vi "PH_PILS.set PPPA.vi"(0 "i ref in":refnum<vi>, 2 "Tagname":string="N/A", 5 "error in":errorcluster) -> (14 "i ref out":refnum<vi>, 19 "error out":errorcluster)   [LabVIEW 2014, in "PH_PILS.lvlib"]
uses:
  PH_PILS.lvlib
  PH_Basics/PH_PP_Common/PH_PP_Common.PUs.ctl
  PH_Basics/PH_PP_Common/PH_PP_Common.PSU Tags.ctl
  PH_Devices/PH_Beckhoff_PP_PU/PH_Beckhoff_PP_PU.RR Tags.ctl
  PH_Basics/PH_Common/PH_Common.lvlib
  PH_Basics/PH_PP_Common/PH_PP_Common.lvlib
  PH_Devices/PH_Beckhoff_PP_PU/PH_Beckhoff_PP_PU.lvlib
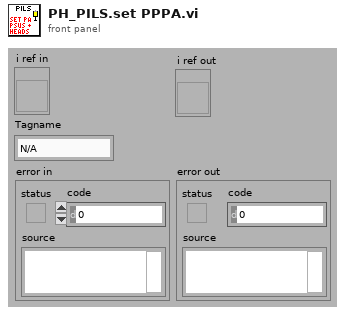
[diagram p1: front panel]
types:
  T1 = typedef "PH_PP_Common.lvlib/PH_PP_Common.PUs.ctl" = enum16{"no Info", "PA-19mm-1", "PA-19mm-2", "PA-45mm-PILC", "PA-45mm-MAIN", "MA-PU-1", "MA-PU-2", "MA-PU-3", "MA-PU-4", "MA-PU-5", "MA-PU-6", "MA-FR", "MA-PILC", "PA-45mm-DP"}
  T2 = typedef "PH_Beckhoff_PP_PU.lvlib/PH_Beckhoff_PP_PU.RR Tags.ctl" = enum16{"open", "closed", "close", "Status"}
  T3 = typedef "PH_PP_Common.lvlib/PH_PP_Common.PSU Tags.ctl" = enum16{"voltage-indicator", "peak-detect", "current", "voltage", "inihibit-indicator", "end-of-charge", "HV-on-indicator", "overtemperature", "interlock-indicator", "load-fault", "sum-fault", "HV-off-indicator", "DC-ok", "inhibit", "HV-on", "interlock", "reset", "Status", "Limits"}
  T4 = typedef "PH_PILS.lvlib/PH_PILS.i attribute.ctl" = cluster{"Boolean":cluster{"GUI Ref":refnum<vi>, "Status":i32}[], "GUI Refs Exp. Shutters":cluster{"1":refnum<vi>, "2":refnum<vi>, "3":refnum<vi>, "4":refnum<vi>}, "Tristate2Run GUI Refs":refnum<vi>[], "EO-Likes":cluster{"GUI Ref":refnum<vi>, "Status":i32}[], "Operation Mode":cluster{"Operation Mode":T5, "GUI":cluster{"Ref State":refnum<vi>, "Ref":refnum<vi>}, "Servicemode":cluster{"Tagname":string, "Status":i32}, "Labormode":cluster{"Tagname":string, "Status":i32}, "Searchmode":cluster{"Tagname":string, "Status":i32}, "Shotmode":cluster{"Tagname":string, "Status":i32}}, "Submode":cluster{"Submode":T6, "GUI":cluster{"Ref State":refnum<vi>, "Ref":refnum<vi>}, "Submode":cluster{"Tagname":string, "Status":i32}}, "Experiment":cluster{"Experiment":enum16{"unknown", "intern", "4 (Z6)", "3", "2", "1"}, "GUI":cluster{"Ref State":refnum<vi>, "Ref":refnum<vi>}, "intern":cluster{"Tagname":string, "Status":i32}, "Exp 4":cluster{"Tagname":string, "Status":i32}, "Exp 3":cluster{"Tagname":string, "Status":i32}, "Exp 2":cluster{"Tagname":string, "Status":i32}, "Exp 1":cluster{"Tagname":string, "Status":i32}}, "TristateNormal":cluster{"GUI Ref":refnum<vi>, "Status":i32}[], "Door Tags":cluster{"GUI Ref":refnum<vi>, "Status":i32}[], "GUIlessTags":cluster{"Name":string, "Status":i32}[], "Beamline GUI Refs":refnum<vi>[], "Special Boolean":cluster{"GUI Ref":refnum<vi>, "Status":i32}[], "Laserpower":cluster{"GUI Ref":refnum<vi>, "Status":i32}[], "Shutter":cluster{"GUI Ref":refnum<vi>, "Status":i32}[], "Tristate EO Like":cluster{"GUI Ref":refnum<vi>, "Status":i32}[], "PP":cluster{"GUI Ref":refnum<vi>, "Status":i32, "Head Ref":refnum<vi>, "Slider Ref":refnum<vi>}[], "Switch Knobs":cluster{"GUI Ref":refnum<vi>, "Status":i32}[], "Latch Knob GUI Refs":refnum<vi>[], "FailureCounter":i32, "Enabled Status":cluster{"Laser":i32, "PreAmp":i32, "MainAmp":i32}, "Mercury":refnum<vi>, "Instance Rods":string, "Logfile":path, "Beckhoff-Instance Internal":string, "Beckhoff-Instance External":string, "Enabling Rights":cluster{"Name":string, "Password":string, "PA?":bool, "MA?":bool, "Exp?":bool}[]}
  T5 = typedef "PH_PILS.lvlib/PH_PILS.Operation Mode.ctl" = enum16{"unknown", "Service", "Labor", "Search", "Shot"}
  T6 = typedef "PH_PILS.lvlib/PH_PILS.Submode.ctl" = enum16{"unknown", "HV-Normal", "HV-Test"}
  T7 = cluster{"GUI Ref":refnum<vi>, "Status":i32, "Head Ref":refnum<vi>, "Slider Ref":refnum<vi>}[]
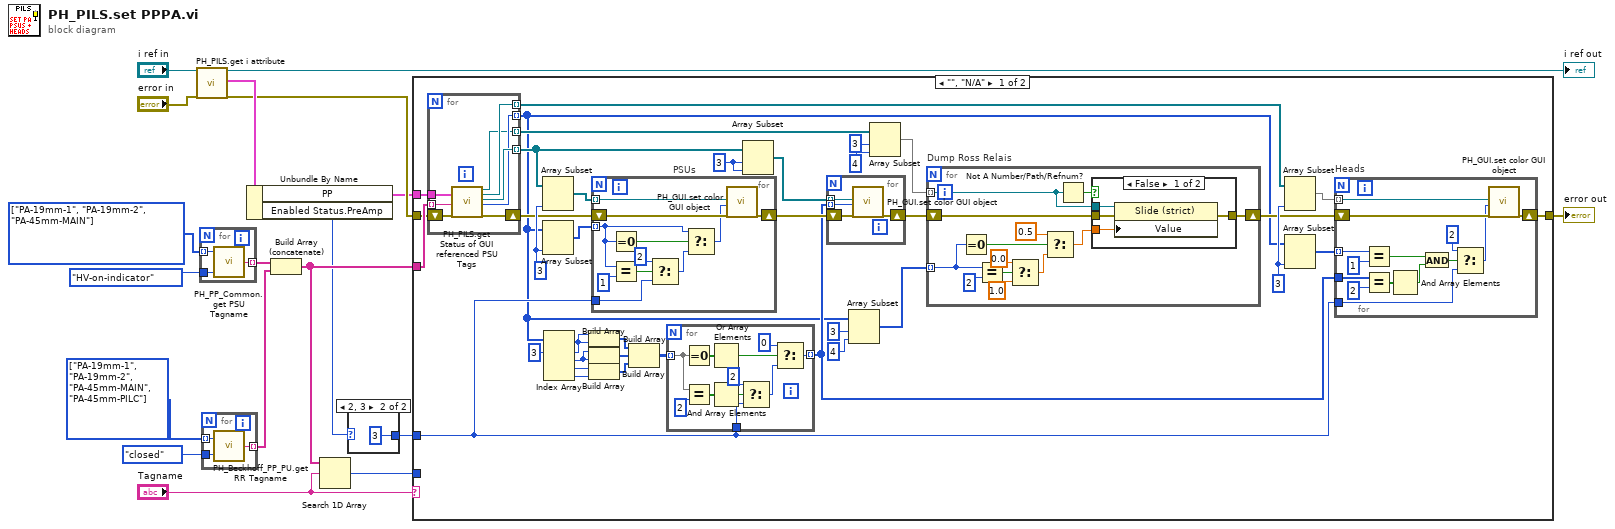
[diagram p0: block diagram]
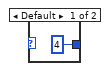
[diagram p2: hidden frame]
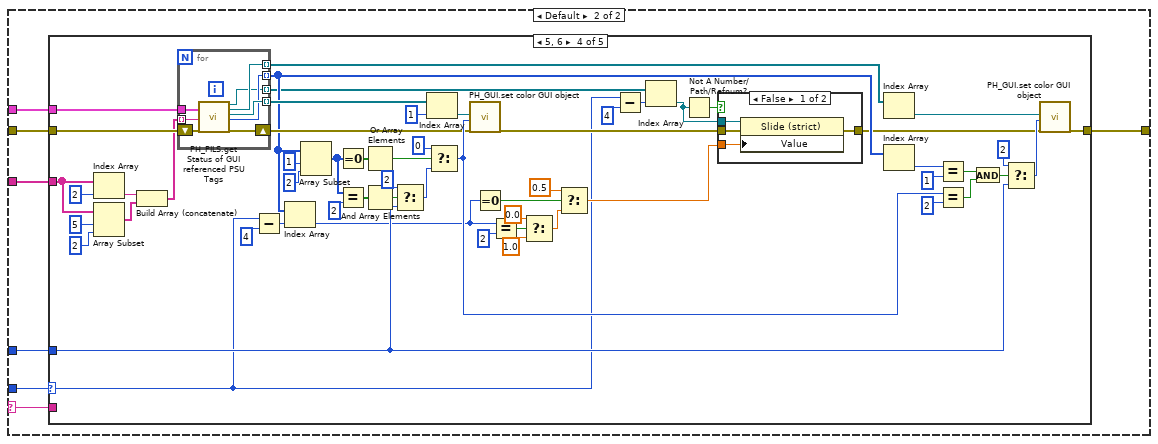
[diagram p4: hidden frame]
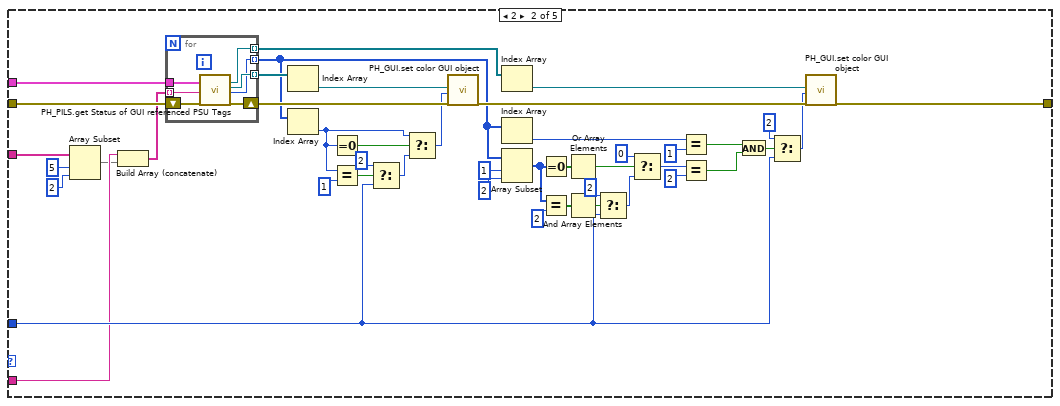
[diagram p6: hidden frame]
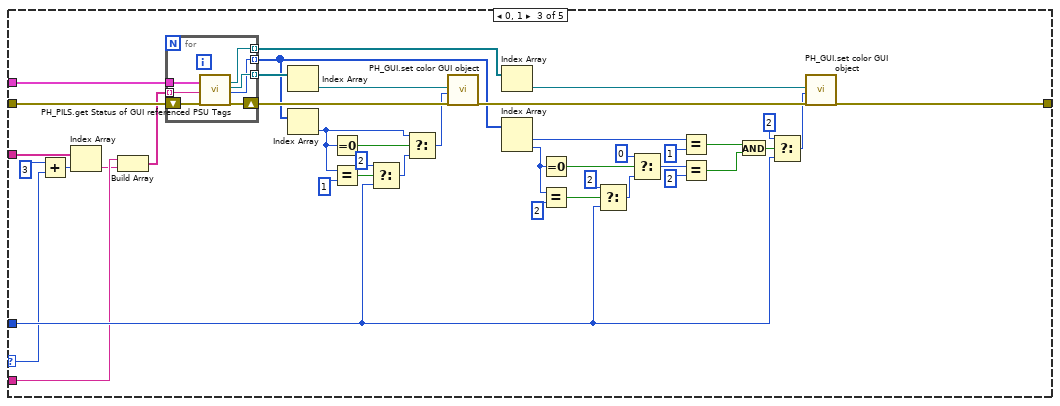
[diagram p7: hidden frame]
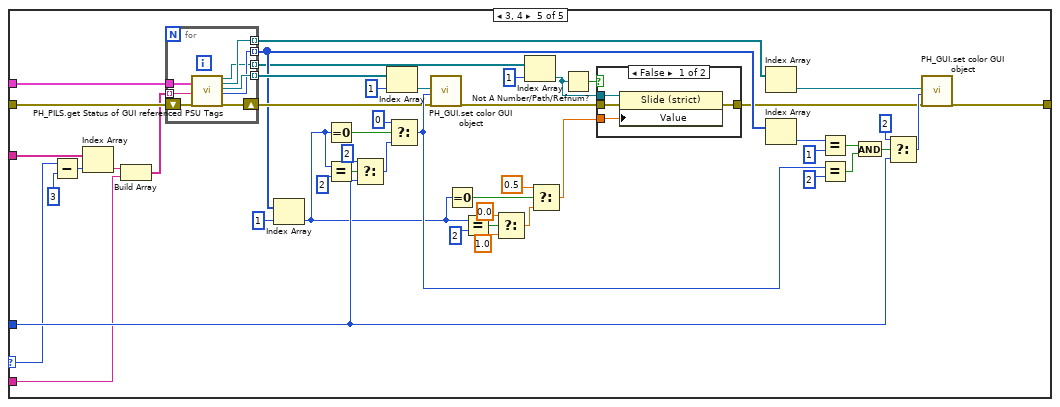
[diagram p9: hidden frame]
diagram:
  w6 = T1[] [enum."PA-19mm-1", enum."PA-19mm-2", enum."PA-45mm-MAIN", enum."PA-45mm-PILC"] items=["no Info", "PA-19mm-1", "PA-19mm-2", "PA-45mm-PILC", "PA-45mm-MAIN", "MA-PU-1", "MA-PU-2", "MA-PU-3", "MA-PU-4", "MA-PU-5", "MA-PU-6", "MA-FR", "MA-PILC", "PA-45mm-DP"]
  w5 = T1[] [enum."PA-19mm-1", enum."PA-19mm-2", enum."PA-45mm-MAIN"] items=["no Info", "PA-19mm-1", "PA-19mm-2", "PA-45mm-PILC", "PA-45mm-MAIN", "MA-PU-1", "MA-PU-2", "MA-PU-3", "MA-PU-4", "MA-PU-5", "MA-PU-6", "MA-FR", "MA-PILC", "PA-45mm-DP"]
  n1 = call "PH_PILS.get i attribute.vi"("i ref in"="i ref in", "error in (no error)"="error in") -> ("i ref out"=→"i ref out":refnum<vi>, "i attribute"=w17:T4, "error out"=w16:errorcluster)  [unwired: 15 in]
  n2 = for {
    tunnel: w5 -> [w21] mode=indexing
    tunnel: PH_PP_Common.PSU_Tags."HV-on-indicator" ("PSU Tag") -> [w20]
    tunnel: [w19] -> w3 mode=indexing
    n3 = call "PH_PP_Common.get PSU Tagname.vi"("PSU Tag"=w20, "PU"=w21) -> ("PSU Tagname"=w19:string)  [unwired: 1 in]
  }
  n4 = for {
    tunnel: w6 -> [w24] mode=indexing
    tunnel: PH_Beckhoff_PP_PU.RR_Tags."closed" ("Ross Relais Tag") -> [w23]
    tunnel: [w22] -> w4 mode=indexing
    n5 = call "PH_Beckhoff_PP_PU.get RR Tagname.vi"("Ross Relais Tag"=w23, "PU"=w24) -> ("RR Tagname"=w22:string)
  }
  n6 = Unbundle By Name(w17) -> ("PP"=w15:T7, "Enabled Status.PreAmp"=w1:i32)
  n7 = Build Array (concatenate)(w3, w4) -> (w8:string[])
  n8 = Search 1D Array(1D array=w8, element="Tagname") -> (index of element=w18:i32)  [unwired: 1 in]
  n9 = case shown="2, 3" w1 {
    tunnel: [4 ("Status") 3 ("Status")] -> w2
    frame Default {
    }
    frame 2, 3 {
    }
  }
  n10 = case shown="\"\", \"N/A\"" "Tagname" {
    selector: "Tagname" -> [_ w131]
    tunnel: w16 -> [w45 w134]
    tunnel: [w63 w136] -> w12
    tunnel: w8 -> [w46 w135]
    tunnel: w18 -> [_ w130]
    tunnel: w15 -> [w44 w133]
    tunnel: w2 -> [w41 w132]
    frame "", "N/A" {
      w43 = 3 ("index")
      w55 = 3 ("length")
      w62 = 3 ("length")
      n11 = for {
        tunnel: w44 -> [w106]
        shift-right: [w110] -> w59
        shift-left: w45 -> [w111]
        tunnel: w46 -> [w105] mode=indexing
        tunnel: [w109] -> w58 mode=indexing
        tunnel: [w108] -> w51 mode=indexing
        tunnel: [w107] -> w28 mode=indexing
        tunnel: [w104] -> w48 mode=indexing
        n12 = call "PH_PILS.get Status of GUI referenced PSU Tags.vi"("PP Tag"=w106, "Tagname"=w105, "error in"=w111) -> ("Slider Ref"=w104:refnum<vi>, "Head Ref"=w109:refnum<vi>, "GUI Ref"=w108:refnum<vi>, "Status"=w107:i32, "error out"=w110:errorcluster)  [unwired: 11 in, 1 out]
      }
      n13 = Array Subset(array=w51, length=w62) -> (w60:refnum<vi>[])  [unwired: 1 in]
      n14 = Array Subset(array=w28, length=w62) -> (w61:i32[])  [unwired: 1 in]
      n15 = Index Array(array=w28, index #1=3 ("index")) -> (element #1=w39:i32, element #2=w38:i32, element #3=w37:i32, element #4=w36:i32)  [unwired: 3 in]
      n16 = Build Array(w39, w39) -> (w33:i32[])
      n17 = Build Array(w38, w38) -> (w34:i32[])
      n18 = Build Array(w37, w36) -> (w35:i32[])
      n19 = for "PSUs" {
        shift-right: [w103] -> w50
        shift-left: w59 -> [w101]
        tunnel: w61 -> [w99] mode=indexing
        tunnel: w60 -> [w102] mode=indexing
        tunnel: w41 -> [w93]
        n20 = Equal To 0?(x=w99) -> (x = 0?=w100:bool)
        n21 = Equal?(x=w99, y=1) -> (x = y?=w97:bool)
        n22 = Select(t=2 ("y"), s=w97, f=w93) -> (s? t:f=w96:i32)
        n23 = Select(t=w99, s=w100, f=w96) -> (s? t:f=w94:i32)
        n24 = call "PH_GUI.set color GUI object.vi"("GUI object Ref"=w102, "State"=w94, "error in (no error)"=w101) -> ("error out"=w103:errorcluster)  [unwired: 16 in]
      }
      n25 = Build Array(w33, w34, w35) -> (w42:i32[][])
      n26 = for {
        tunnel: w42 -> [w66] mode=indexing
        tunnel: [w65] -> w29 mode=indexing
        tunnel: w41 -> [w64]
        n27 = Equal To 0?(x=w66) -> (x = 0?=w74:bool[])
        n28 = Equal?(x=w66, y=2) -> (x = y?=w71:bool[])
        n29 = Or Array Elements(Boolean array=w74) -> (logical OR=w73:bool)
        n30 = And Array Elements(Boolean array=w71) -> (logical AND=w69:bool)
        n31 = Select(t=2 ("State"), s=w69, f=w64) -> (s? t:f=w68:i32)
        n32 = Select(t=0 ("State"), s=w73, f=w68) -> (s? t:f=w65:i32)
      }
      n33 = Array Subset(array=w51, index=w43, length=w43) -> (w54:refnum<vi>[])
      n34 = for {
        tunnel: w54 -> [w78] mode=indexing
        shift-right: [w76] -> w49
        shift-left: w50 -> [w77]
        tunnel: w29 -> [w75] mode=indexing
        n35 = call "PH_GUI.set color GUI object.vi"("GUI object Ref"=w78, "State"=w75, "error in (no error)"=w77) -> ("error out"=w76:errorcluster)  [unwired: 16 in]
      }
      n36 = Array Subset(array=w28, index=3, length=4) -> (w30:i32[])
      n37 = Array Subset(array=w48, index=3, length=4) -> (w27:refnum<vi>[])
      n38 = for "Dump Ross Relais" {
        shift-right: [w123] -> w47
        shift-left: w49 -> [w113]
        tunnel: w27 -> [w124] mode=indexing
        tunnel: w30 -> [w114] mode=indexing
        n39 = Equal To 0?(x=w114) -> (x = 0?=w122:bool)
        n40 = Equal?(x=w114, y=2) -> (x = y?=w118:bool)
        n41 = Select(t=0.0, s=w118, f=1.0) -> (s? t:f=w117:dbl)
        n42 = Select(t=0.5, s=w122, f=w117) -> (s? t:f=w121:dbl)
        n43 = Not A Number/Path/Refnum?(number/path/refnum=w124) -> (NaN/Path/Refnum?=w112:bool)
        n44 = case shown="False" w112 {
          tunnel: w113 -> [w126 w129]
          tunnel: [w128 w129] -> w123
          tunnel: w121 -> [w127 _]
          tunnel: w124 -> [w125 _]
          frame False {
            n45 = property class="Slide (strict)"(reference=w125, error in=w126, "Value"=w127) -> (error out=w128:errorcluster)  [unwired: 1 out]
          }
          frame True {
          }
        }
      }
      n46 = Array Subset(array=w58, length=w55) -> (w57:refnum<vi>[])  [unwired: 1 in]
      n47 = Array Subset(array=w28, length=w55) -> (w56:i32[])  [unwired: 1 in]
      n48 = for "Heads" {
        shift-right: [w92] -> w63
        shift-left: w47 -> [w89]
        tunnel: w57 -> [w91] mode=indexing
        tunnel: w56 -> [w90] mode=indexing
        tunnel: w29 -> [w88]
        tunnel: w41 -> [w82]
        n49 = Equal?(x=w90, y=1) -> (x = y?=w80:bool)
        n50 = Equal?(x=w88, y=2 ("Status")) -> (x = y?=w86:bool[])
        n51 = And Array Elements(Boolean array=w86) -> (logical AND=w79:bool)
        n52 = And(x=w80, y=w79) -> (x .and. y?=w85:bool)
        n53 = Select(t=2 ("Status"), s=w85, f=w82) -> (s? t:f=w83:i32)
        n54 = call "PH_GUI.set color GUI object.vi"("GUI object Ref"=w91, "State"=w83, "error in (no error)"=w89) -> ("error out"=w92:errorcluster)  [unwired: 16 in]
      }
    }
    frame Default {
      n55 = case shown="5, 6" w130 {
        selector: w130 -> [_ _ w193 w237 w327]
        tunnel: [w137 w181 w229 w293 w355] -> w136
        tunnel: w135 -> [_ w167 w196 w283 w326]
        tunnel: w134 -> [w137 w173 w221 w289 w351]
        tunnel: w133 -> [_ w172 w220 w288 w350]
        tunnel: w132 -> [_ w171 w219 w287 w349]
        tunnel: w131 -> [_ w169 w217 _ w324]
        frame Default {
        }
        frame 2 {
          n56 = Array Subset(array=w167, index=5, length=2) -> (w164:string[])
          n57 = Build Array (concatenate)(w169, w164) -> (w168:string[])
          n58 = for {
            tunnel: w172 -> [w182]
            shift-right: [w187] -> w178
            shift-left: w173 -> [w188]
            tunnel: w168 -> [w183] mode=indexing
            tunnel: [w186] -> w177 mode=indexing
            tunnel: [w185] -> w174 mode=indexing
            tunnel: [w184] -> w155 mode=indexing
            n59 = call "PH_PILS.get Status of GUI referenced PSU Tags.vi"("PP Tag"=w182, "Tagname"=w183, "error in"=w188) -> ("Head Ref"=w186:refnum<vi>, "GUI Ref"=w185:refnum<vi>, "Status"=w184:i32, "error out"=w187:errorcluster)  [unwired: 11 in, 2 out]
          }
          n60 = Index Array(array=w174) -> (element=w179:refnum<vi>)  [unwired: 1 in]
          n61 = Index Array(array=w155) -> (element=w180:i32)  [unwired: 1 in]
          n62 = Equal To 0?(x=w180) -> (x = 0?=w163:bool)
          n63 = Equal?(x=w180, y=1) -> (x = y?=w161:bool)
          n64 = Select(t=2 ("y"), s=w161, f=w171) -> (s? t:f=w160:i32)
          n65 = Select(t=w180, s=w163, f=w160) -> (s? t:f=w158:i32)
          n66 = call "PH_GUI.set color GUI object.vi"("GUI object Ref"=w179, "State"=w158, "error in (no error)"=w178) -> ("error out"=w170:errorcluster)  [unwired: 16 in]
          n67 = Index Array(array=w177) -> (element=w176:refnum<vi>)  [unwired: 1 in]
          n68 = Index Array(array=w155) -> (element=w175:i32)  [unwired: 1 in]
          n69 = Array Subset(array=w155, index=1, length=2) -> (w153:i32[])
          n70 = Equal To 0?(x=w153) -> (x = 0?=w152:bool[])
          n71 = Equal?(x=w153, y=2) -> (x = y?=w149:bool[])
          n72 = Or Array Elements(Boolean array=w152) -> (logical OR=w151:bool)
          n73 = And Array Elements(Boolean array=w149) -> (logical AND=w147:bool)
          n74 = Select(t=2 ("State"), s=w147, f=w171) -> (s? t:f=w146:i32)
          n75 = Select(t=0 ("State"), s=w151, f=w146) -> (s? t:f=w154:i32)
          n76 = Equal?(x=w175, y=1) -> (x = y?=w139:bool)
          n77 = Equal?(x=w154, y=2 ("Status")) -> (x = y?=w138:bool)
          n78 = And(x=w139, y=w138) -> (x .and. y?=w143:bool)
          n79 = Select(t=2 ("Status"), s=w143, f=w171) -> (s? t:f=w141:i32)
          n80 = call "PH_GUI.set color GUI object.vi"("GUI object Ref"=w176, "State"=w141, "error in (no error)"=w170) -> ("error out"=w181:errorcluster)  [unwired: 16 in]
        }
        frame 0, 1 {
          n81 = Add(x=3, y=w193) -> (x+y=w194:i32)
          n82 = Index Array(array=w196, index=w194) -> (element=w195:string)
          n83 = Build Array(w217, w195) -> (w216:string[])
          n84 = for {
            tunnel: w220 -> [w230]
            shift-right: [w235] -> w226
            shift-left: w221 -> [w236]
            tunnel: w216 -> [w231] mode=indexing
            tunnel: [w234] -> w225 mode=indexing
            tunnel: [w233] -> w222 mode=indexing
            tunnel: [w232] -> w209 mode=indexing
            n85 = call "PH_PILS.get Status of GUI referenced PSU Tags.vi"("PP Tag"=w230, "Tagname"=w231, "error in"=w236) -> ("Head Ref"=w234:refnum<vi>, "GUI Ref"=w233:refnum<vi>, "Status"=w232:i32, "error out"=w235:errorcluster)  [unwired: 11 in, 2 out]
          }
          n86 = Index Array(array=w222) -> (element=w227:refnum<vi>)  [unwired: 1 in]
          n87 = Index Array(array=w209) -> (element=w228:i32)  [unwired: 1 in]
          n88 = Equal To 0?(x=w228) -> (x = 0?=w215:bool)
          n89 = Equal?(x=w228, y=1) -> (x = y?=w213:bool)
          n90 = Select(t=2 ("y"), s=w213, f=w219) -> (s? t:f=w212:i32)
          n91 = Select(t=w228, s=w215, f=w212) -> (s? t:f=w210:i32)
          n92 = call "PH_GUI.set color GUI object.vi"("GUI object Ref"=w227, "State"=w210, "error in (no error)"=w226) -> ("error out"=w218:errorcluster)  [unwired: 16 in]
          n93 = Index Array(array=w225) -> (element=w224:refnum<vi>)  [unwired: 1 in]
          n94 = Index Array(array=w209) -> (element #1=w223:i32, element #2=w189:i32)  [unwired: 2 in]
          n95 = Equal To 0?(x=w189) -> (x = 0?=w190:bool)
          n96 = Equal?(x=w189, y=2) -> (x = y?=w191:bool)
          n97 = Select(t=2 ("State"), s=w191, f=w219) -> (s? t:f=w205:i32)
          n98 = Select(t=0 ("State"), s=w190, f=w205) -> (s? t:f=w208:i32)
          n99 = Equal?(x=w223, y=1) -> (x = y?=w198:bool)
          n100 = Equal?(x=w208, y=2 ("Status")) -> (x = y?=w197:bool)
          n101 = And(x=w198, y=w197) -> (x .and. y?=w202:bool)
          n102 = Select(t=2 ("Status"), s=w202, f=w219) -> (s? t:f=w200:i32)
          n103 = call "PH_GUI.set color GUI object.vi"("GUI object Ref"=w224, "State"=w200, "error in (no error)"=w218) -> ("error out"=w229:errorcluster)  [unwired: 16 in]
        }
        frame 5, 6 {
          n104 = Index Array(array=w283, index=2) -> (element=w280:string)
          n105 = Array Subset(array=w283, index=5, length=2) -> (w279:string[])
          n106 = Build Array (concatenate)(w280, w279) -> (w278:string[])
          n107 = for {
            tunnel: w288 -> [w300]
            shift-right: [w305] -> w285
            shift-left: w289 -> [w306]
            tunnel: w278 -> [w301] mode=indexing
            tunnel: [w304] -> w292 mode=indexing
            tunnel: [w303] -> w277 mode=indexing
            tunnel: [w302] -> w256 mode=indexing
            tunnel: [w299] -> w248 mode=indexing
            n108 = call "PH_PILS.get Status of GUI referenced PSU Tags.vi"("PP Tag"=w300, "Tagname"=w301, "error in"=w306) -> ("Slider Ref"=w299:refnum<vi>, "Head Ref"=w304:refnum<vi>, "GUI Ref"=w303:refnum<vi>, "Status"=w302:i32, "error out"=w305:errorcluster)  [unwired: 11 in, 1 out]
          }
          n109 = Subtract(x=w237, y=4) -> (x-y=w255:i32)
          n110 = Index Array(array=w256, index=w255) -> (element=w251:i32)
          n111 = Array Subset(array=w256, index=1, length=2) -> (w272:i32[])
          n112 = Equal To 0?(x=w272) -> (x = 0?=w271:bool[])
          n113 = Equal?(x=w272, y=2) -> (x = y?=w268:bool[])
          n114 = Or Array Elements(Boolean array=w271) -> (logical OR=w270:bool)
          n115 = And Array Elements(Boolean array=w268) -> (logical AND=w266:bool)
          n116 = Select(t=2 ("State"), s=w266, f=w287) -> (s? t:f=w265:i32)
          n117 = Index Array(array=w277, index=1) -> (element=w275:refnum<vi>)
          n118 = Select(t=0 ("State"), s=w270, f=w265) -> (s? t:f=w286:i32)
          n119 = call "PH_GUI.set color GUI object.vi"("GUI object Ref"=w275, "State"=w286, "error in (no error)"=w285) -> ("error out"=w253:errorcluster)  [unwired: 16 in]
          n120 = Equal To 0?(x=w251) -> (x = 0?=w246:bool)
          n121 = Equal?(x=w251, y=2) -> (x = y?=w242:bool)
          n122 = Select(t=0.0, s=w242, f=1.0) -> (s? t:f=w241:dbl)
          n123 = Select(t=0.5, s=w246, f=w241) -> (s? t:f=w245:dbl)
          n124 = Subtract(x=w237, y=4) -> (x-y=w250:i32)
          n125 = Index Array(array=w248, index=w250) -> (element=w247:refnum<vi>)
          n126 = Not A Number/Path/Refnum?(number/path/refnum=w247) -> (NaN/Path/Refnum?=w238:bool)
          n127 = case shown="False" w238 {
            tunnel: w253 -> [w295 w298]
            tunnel: [w297 w298] -> w252
            tunnel: w245 -> [w296 _]
            tunnel: w247 -> [w294 _]
            frame False {
              n128 = property class="Slide (strict)"(reference=w294, error in=w295, "Value"=w296) -> (error out=w297:errorcluster)  [unwired: 1 out]
            }
            frame True {
            }
          }
          n129 = Index Array(array=w292) -> (element=w291:refnum<vi>)  [unwired: 1 in]
          n130 = Index Array(array=w256) -> (element=w290:i32)  [unwired: 1 in]
          n131 = Equal?(x=w290, y=1) -> (x = y?=w258:bool)
          n132 = Equal?(x=w286, y=2 ("Status")) -> (x = y?=w257:bool)
          n133 = And(x=w258, y=w257) -> (x .and. y?=w262:bool)
          n134 = Select(t=2 ("Status"), s=w262, f=w287) -> (s? t:f=w260:i32)
          n135 = call "PH_GUI.set color GUI object.vi"("GUI object Ref"=w291, "State"=w260, "error in (no error)"=w252) -> ("error out"=w293:errorcluster)  [unwired: 16 in]
        }
        frame 3, 4 {
          n136 = Subtract(x=w327, y=3) -> (x-y=w330:i32)
          n137 = Index Array(array=w326, index=w330) -> (element=w325:string)
          n138 = Build Array(w325, w324) -> (w346:string[])
          n139 = for {
            tunnel: w350 -> [w361]
            shift-right: [w367] -> w347
            shift-left: w351 -> [w368]
            tunnel: w346 -> [w363] mode=indexing
            tunnel: [w366] -> w354 mode=indexing
            tunnel: [w365] -> w345 mode=indexing
            tunnel: [w364] -> w331 mode=indexing
            tunnel: [w362] -> w311 mode=indexing
            n140 = call "PH_PILS.get Status of GUI referenced PSU Tags.vi"("PP Tag"=w361, "Tagname"=w363, "error in"=w368) -> ("Slider Ref"=w362:refnum<vi>, "Head Ref"=w366:refnum<vi>, "GUI Ref"=w365:refnum<vi>, "Status"=w364:i32, "error out"=w367:errorcluster)  [unwired: 11 in, 1 out]
          }
          n141 = Index Array(array=w331, index=1) -> (element=w309:i32)
          n142 = Equal To 0?(x=w309) -> (x = 0?=w323:bool)
          n143 = Equal?(x=w309, y=2) -> (x = y?=w322:bool)
          n144 = Select(t=2 ("State"), s=w322, f=w349) -> (s? t:f=w340:i32)
          n145 = Index Array(array=w345, index=1) -> (element=w343:refnum<vi>)
          n146 = Select(t=0 ("State"), s=w323, f=w340) -> (s? t:f=w348:i32)
          n147 = call "PH_GUI.set color GUI object.vi"("GUI object Ref"=w343, "State"=w348, "error in (no error)"=w347) -> ("error out"=w308:errorcluster)  [unwired: 16 in]
          n148 = Equal To 0?(x=w309) -> (x = 0?=w321:bool)
          n149 = Equal?(x=w309, y=2) -> (x = y?=w317:bool)
          n150 = Select(t=0.0, s=w317, f=1.0) -> (s? t:f=w316:dbl)
          n151 = Index Array(array=w311, index=1) -> (element=w310:refnum<vi>)
          n152 = Select(t=0.5, s=w321, f=w316) -> (s? t:f=w320:dbl)
          n153 = Not A Number/Path/Refnum?(number/path/refnum=w310) -> (NaN/Path/Refnum?=w313:bool)
          n154 = case shown="False" w313 {
            tunnel: w308 -> [w357 w360]
            tunnel: [w359 w360] -> w307
            tunnel: w320 -> [w358 _]
            tunnel: w310 -> [w356 _]
            frame False {
              n155 = property class="Slide (strict)"(reference=w356, error in=w357, "Value"=w358) -> (error out=w359:errorcluster)  [unwired: 1 out]
            }
            frame True {
            }
          }
          n156 = Index Array(array=w354) -> (element=w353:refnum<vi>)  [unwired: 1 in]
          n157 = Index Array(array=w331) -> (element=w352:i32)  [unwired: 1 in]
          n158 = Equal?(x=w352, y=1) -> (x = y?=w333:bool)
          n159 = Equal?(x=w348, y=2 ("Status")) -> (x = y?=w332:bool)
          n160 = And(x=w333, y=w332) -> (x .and. y?=w337:bool)
          n161 = Select(t=2 ("Status"), s=w337, f=w349) -> (s? t:f=w335:i32)
          n162 = call "PH_GUI.set color GUI object.vi"("GUI object Ref"=w353, "State"=w335, "error in (no error)"=w307) -> ("error out"=w355:errorcluster)  [unwired: 16 in]
        }
      }
    }
  }
  "error out" <- w12
